vi "LED1.vi"(11 "LED1":bool) -> ()   [LabVIEW 2021]
uses:
  <vilib>/rvi/eio/common/nirviEmuTemplateMethod_errors.vi
  <vilib>/eio/EIONode/EIONode.xnode
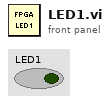
[diagram p1: front panel]
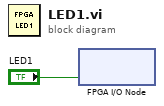
[diagram p0: block diagram]
diagram:
  n1 = xnode "FPGA I/O Node"("LED1"="LED1") -> ()  [unwired: 1 in, 1 out]
